vi "CRYInsert Result.vi"(8 "sOptionUpdate":string, 9 "sOption":string, 10 "Index":i32[](array[numeric]), 11 "Result":T1 {"Margin" format="%.2f"}) -> (2 "Inserted Index":i32[](array[numeric]), 3 "Inserted Name Out":string[](array[string]))   [LabVIEW 2013]
uses:
  CRYSystem/Typedef Control/CRYResult Cluster Array.ctl
  CRYSystem/Typedef Control/CRYResult Cluster.ctl
  Global/CRYCurve Library Global.vi
  Global/CRYCurves Array Global.vi
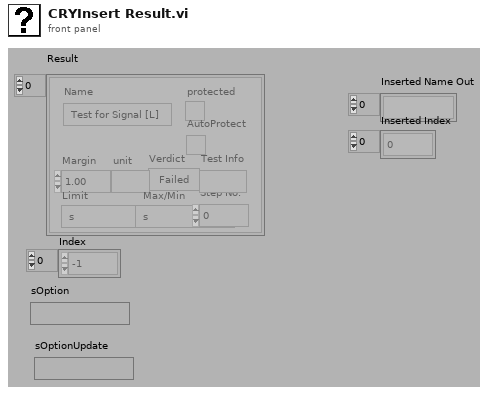
[diagram p1: front panel]
types:
  T1 = typedef "CRYResult Cluster Array.ctl" = T2[]
  T2 = typedef "CRYResult Cluster.ctl" = cluster{"Name":string, "Margin":dbl, "unit":string, "Verdict":bool, "Limit":string, "Max/Min":string, "protected":bool, "Step No.":i32, "Test Info":string, "AutoProtect":bool}
  T3 = cluster{"CurveOld":string[], "ValueOld":string[], "ResultOld":string[], "WFMOld":string[], "CurveNew":string[], "ValueNew":string[], "ResultNew":string[], "WFMNew":string[]}
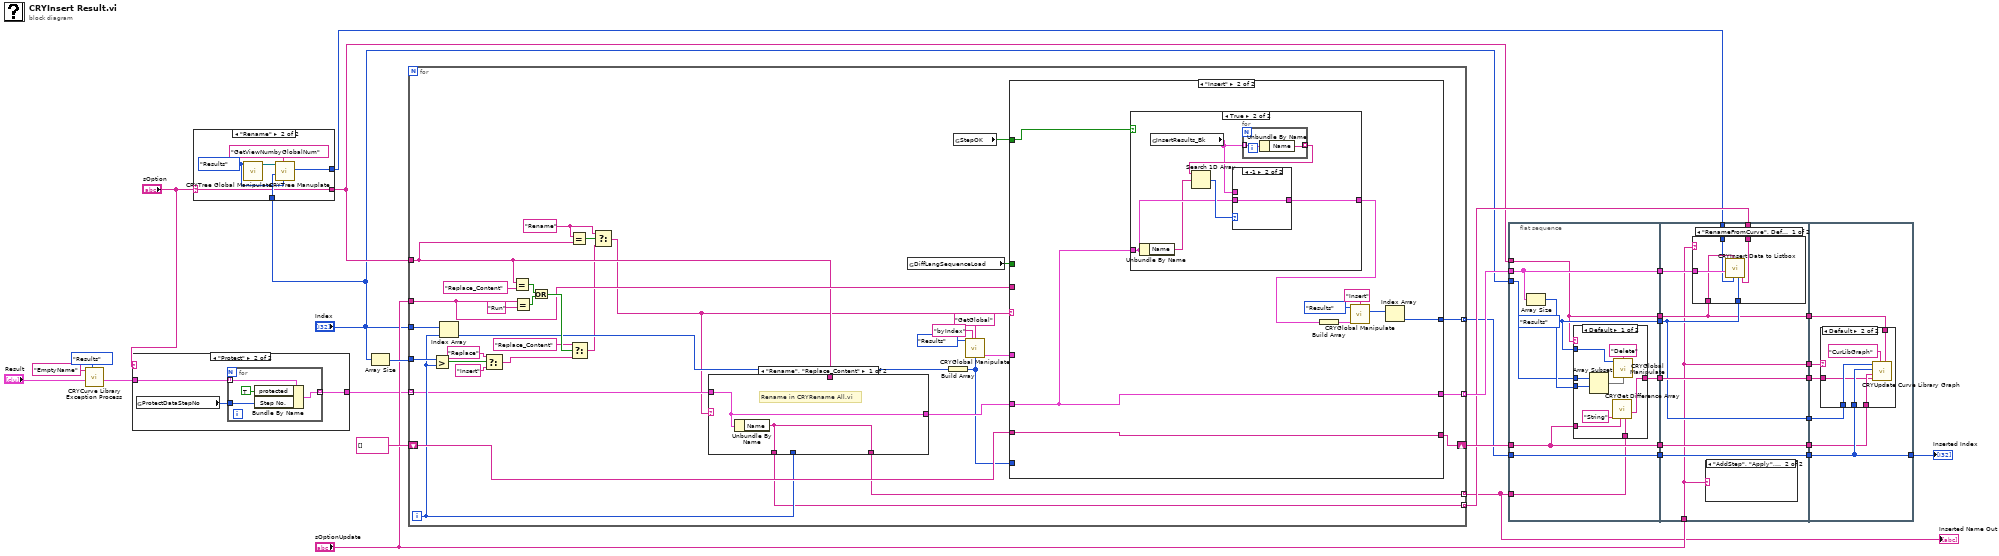
[diagram p0: block diagram]
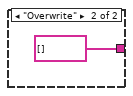
[diagram p4: hidden frame]
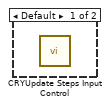
[diagram p5: hidden frame]
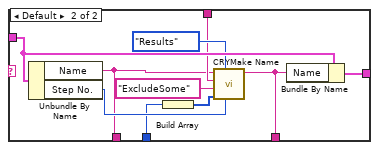
[diagram p8: hidden frame]
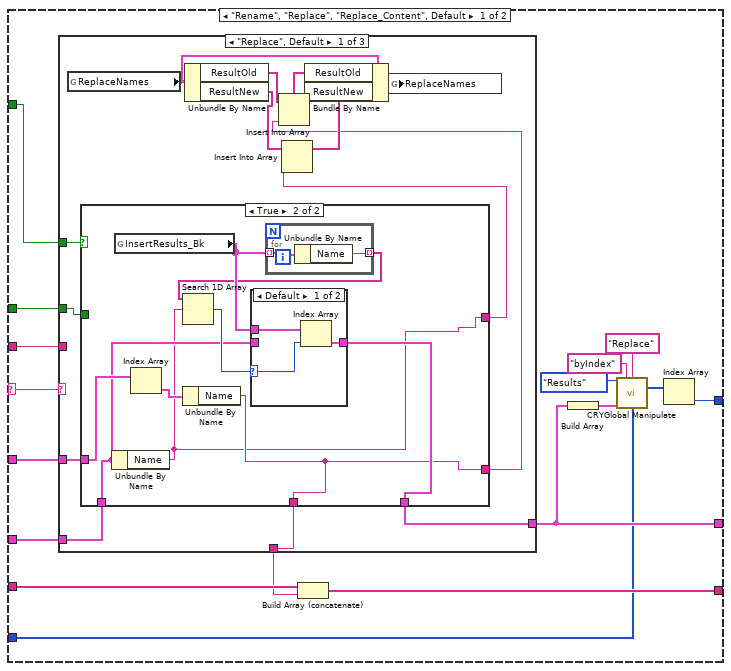
[diagram p9: hidden frame]
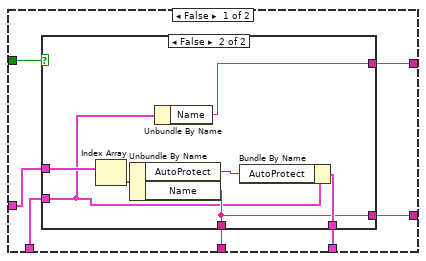
[diagram p10: hidden frame]
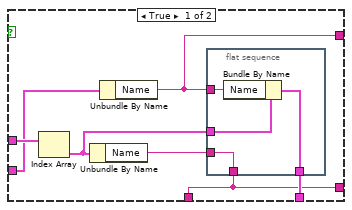
[diagram p11: hidden frame]
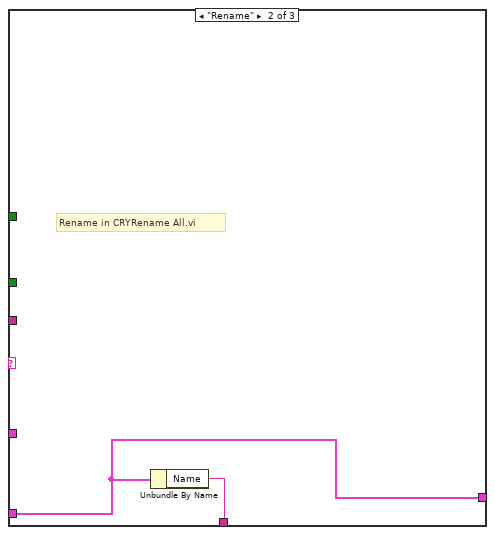
[diagram p13: hidden frame]
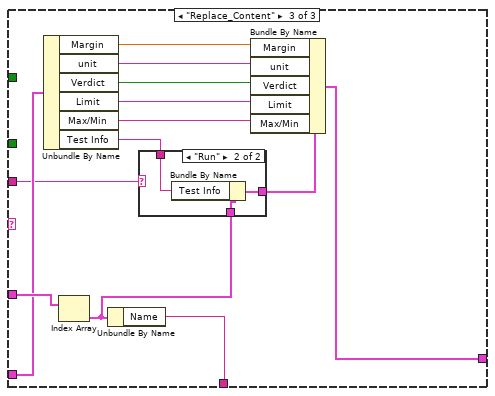
[diagram p14: hidden frame]
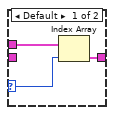
[diagram p17: hidden frame]
diagram:
  n1 = call "CRYCurve Library Exception Process.vi"("Type In"=enum16{"Curves", "Values", "Results", "WFM"}."Results", "Result"="Result", "sAction"="EmptyName") -> ("Result Out"=w1:T1)  [unwired: 6 in, 2 out]
  n2 = case shown="\"Protect\"" "sOption" {
    tunnel: w1 -> [w31 w34]
    tunnel: [w31 w33] -> w7
    frame Default {
    }
    frame "Protect" {
      n3 = global read "CRYCurve Library Global.vi" "ProtectDataStepNo"() -> (w32:i32)
      n4 = for {
        tunnel: w34 -> [w38] mode=indexing
        tunnel: [w37] -> w33 mode=indexing
        tunnel: w32 -> [w35]
        n5 = Bundle By Name(cluster=w38, "protected"=TRUE, "Step No."=w35) -> (w37:T2)
      }
    }
  }
  n6 = case shown="\"Rename\"" "sOption" {
    selector: "sOption" -> [w39 w41]
    tunnel: "Index" -> [_ w42]
    tunnel: [_ w43] -> w9
    tunnel: [w39 w41] -> w11
    frame Default {
    }
    frame "Rename" {
      w40 = enum16{"Curves", "Values", "Results", "WFM"}."Results" ("Type In")
      n7 = call "CRYTree Global Manipulate.vi"("Type In"=w40) -> ("Tree/Curve Tree"=w44:refnum<vi>)  [unwired: 7 in, 3 out]
      n8 = call "CRYTree Manuplate.vi"("Type"=w40, "sAction"="GetViewNumbyGlobalNum", "nData"=w42, "Tree in"=w44) -> ("nData Out"=w43:i32[])  [unwired: 4 in, 3 out]
    }
  }
  n9 = Array Size(array="Index") -> (size(s)=w18:i32)
  n10 = for {
    tunnel: [w71] -> w5 mode=indexing
    tunnel: "Index" -> [w70]
    tunnel: w7 -> [w61] mode=indexing
    tunnel: [w76] -> w29 mode=indexing
    tunnel: w18 -> [w79]
    shift-right: [w77] -> w28
    shift-left: string[] [] -> [w78]
    tunnel: w11 -> [w51]
    tunnel: "sOptionUpdate" -> [w62]
    tunnel: [w54] -> w12 mode=indexing
    tunnel: [w47] -> w6 mode=indexing
    i -> [w69]
    w53 = "Rename" ("y")
    n11 = Greater?(x=w79, y=w69) -> (0:w73:bool)
    n12 = Index Array(array=w70, index=w69) -> (element=w56:i32)
    n13 = Select(t="Replace" ("sOption"), s=w73, f="Insert" ("sOption")) -> (s? t:f=w72:string)
    n14 = Equal?(x=w51, y="Replace_Content") -> (x = y?=w66:bool)
    n15 = Equal?(x=w62, y="Run") -> (x = y?=w65:bool)
    n16 = Or(x=w66, y=w65) -> (x .or. y?=w64:bool)
    n17 = Equal?(x=w53, y=w51) -> (x = y?=w52:bool)
    n18 = Select(t="Replace_Content" ("y"), s=w64, f=w72) -> (s? t:f=w50:string)
    n19 = Select(t=w53, s=w52, f=w50) -> (s? t:f=w49:string)
    n20 = case shown="\"Rename\", \"Replace_Content\"" w49 {
      tunnel: [w82 w92] -> w80
      tunnel: w61 -> [w82 w91]
      tunnel: [w81 w90] -> w71
      tunnel: w69 -> [_ w85]
      tunnel: w51 -> [_ w84]
      tunnel: [w81 w83] -> w54
      frame "Rename", "Replace_Content" {
        # "Rename in CRYRename All.vi"
        n21 = Unbundle By Name(w82) -> ("Name"=w81:string)
      }
      frame Default {
        n22 = Unbundle By Name(w91) -> ("Name"=w83:string, "Step No."=w86:i32)
        n23 = Build Array(w85) -> (w88:i32[])
        n24 = call "CRYMake Name.vi"("Step No."=w86, "Type"=enum16{"Curves", "Values", "Results", "WFM"}."Results", "nData"=w88, "sOption"="ExcludeSome", "sAction"=w84, "Name In"=w83) -> ("Name Out"=w90:string)  [unwired: 4 in, 1 out]
        n25 = Bundle By Name(cluster=w91, "Name"=w90) -> (w92:T2)
      }
    }
    n26 = global read "CRYCurve Library Global.vi" "DiffLangSequenceLoad"() -> (w48:bool)
    n27 = Build Array(w56) -> (w57:i32[])
    n28 = global read "CRYCurve Library Global.vi" "StepOK"() -> (w46:bool)
    n29 = call "CRYGlobal Manipulate.vi"("Type"=enum16{"Curves", "Values", "Results", "WFM"}."Results", "sOption"="byIndex", "sAction"="GetGlobal", "nData"=w57) -> ("Results Out"=w60:T2[])  [unwired: 5 in, 6 out]
    n30 = case shown="\"Insert\"" w49 {
      selector: w49 -> [w104 _]
      tunnel: w60 -> [w108 _]
      tunnel: w80 -> [w109 w184]
      tunnel: [w106 w191] -> w77
      tunnel: w78 -> [w107 w191]
      tunnel: [w100 w184] -> w76
      tunnel: w62 -> [w103 _]
      tunnel: w57 -> [w98 _]
      tunnel: w48 -> [w96 _]
      tunnel: [w94 w186] -> w47
      tunnel: w46 -> [w93 w185]
      frame "Rename", "Replace", "Replace_Content", Default {
        n31 = case shown="\"Replace\", Default" w104 {
          tunnel: w109 -> [w119 w164 w175]
          tunnel: w108 -> [w123 _ w178]
          tunnel: [w122 w165 w177] -> w105
          tunnel: [w121 w164 w176] -> w100
          tunnel: w103 -> [_ _ w169]
          tunnel: w96 -> [w120 _ _]
          tunnel: w93 -> [w110 _ _]
          frame "Replace", Default {
            n32 = global read "CRYCurve Library Global.vi" "ReplaceNames"() -> (w118:T3)
            n33 = case shown="True" w110 {
              tunnel: w123 -> [w130 w153]
              tunnel: [w129 w150] -> w122
              tunnel: [w128 w151] -> w121
              tunnel: w120 -> [w127 _]
              tunnel: w119 -> [w126 w152]
              tunnel: [w125 w149] -> w112
              tunnel: [w124 w150] -> w111
              frame False {
                n34 = case shown="False" w127 {
                  tunnel: w130 -> [w137 w147]
                  tunnel: [w132 w143] -> w129
                  tunnel: [w136 w145] -> w128
                  tunnel: w126 -> [w135 w142]
                  tunnel: [w132 w143] -> w124
                  tunnel: [w131 w144] -> w125
                  frame True {
                    n35 = Index Array(array=w137) -> (element=w134:T2)  [unwired: 1 in]
                    n36 = Unbundle By Name(w134) -> ("Name"=w133:string)
                    n37 = Unbundle By Name(w135) -> ("Name"=w131:string)
                    n38 = flat-sequence {
                      tunnel: [w141] -> w136
                      tunnel: w134 -> [w140]
                      tunnel: w131 -> [w139]
                      tunnel: w133 -> [w138]
                      tunnel: [w138] -> w132
                      frame #0 {
                        n39 = Bundle By Name(cluster=w140, "Name"=w139) -> (w141:T2)
                      }
                    }
                  }
                  frame False {
                    n40 = Index Array(array=w147) -> (element=w148:T2)  [unwired: 1 in]
                    n41 = Unbundle By Name(w148) -> ("AutoProtect"=w146:bool, "Name"=w143:string)
                    n42 = Unbundle By Name(w142) -> ("Name"=w144:string)
                    n43 = Bundle By Name(cluster=w142, "AutoProtect"=w146) -> (w145:T2)
                  }
                }
              }
              frame True {
                n44 = Unbundle By Name(w152) -> ("Name"=w149:string)
                n45 = global read "CRYCurves Array Global.vi" "InsertResults_Bk"() -> (w156:T1)
                n46 = Index Array(array=w153) -> (element=w157:T2)  [unwired: 1 in]
                n47 = Unbundle By Name(w157) -> ("Name"=w150:string)
                n48 = for {
                  tunnel: w156 -> [w163] mode=indexing
                  tunnel: [w162] -> w154 mode=indexing
                  n49 = Unbundle By Name(w163) -> ("Name"=w162:string)
                }
                n50 = Search 1D Array(1D array=w154, element=w149) -> (index of element=w155:i32)  [unwired: 1 in]
                n51 = case shown="Default" w155 {
                  selector: w155 -> [w159 _]
                  tunnel: w156 -> [w160 _]
                  tunnel: [w158 w161] -> w151
                  tunnel: w152 -> [_ w161]
                  frame Default {
                    n52 = Index Array(array=w160, index=w159) -> (element=w158:T2)
                  }
                  frame -1 {
                  }
                }
              }
            }
            n53 = Unbundle By Name(w118) -> ("ResultOld"=w116:string[], "ResultNew"=w115:string[])
            n54 = Insert Into Array(array=w116, new element=w111) -> (w114:string[])  [unwired: 1 in]
            n55 = Insert Into Array(array=w115, new element=w112) -> (w113:string[])  [unwired: 1 in]
            n56 = Bundle By Name(cluster=w118, "ResultOld"=w114, "ResultNew"=w113) -> (w117:T3)
            n57 = global write "CRYCurve Library Global.vi" "ReplaceNames"(w117) -> ()
          }
          frame "Rename" {
            # "Rename in CRYRename All.vi"
            n58 = Unbundle By Name(w164) -> ("Name"=w165:string)
          }
          frame "Replace_Content" {
            n59 = Unbundle By Name(w175) -> ("Margin"=w174:dbl, "unit"=w173:string, "Verdict"=w172:bool, "Limit"=w171:string, "Max/Min"=w170:string, "Test Info"=w168:string)
            n60 = Index Array(array=w178) -> (element=w167:T2)  [unwired: 1 in]
            n61 = Unbundle By Name(w167) -> ("Name"=w177:string)
            n62 = case shown="\"Run\"" w169 {
              tunnel: w167 -> [w179 w182]
              tunnel: [w179 w181] -> w166
              tunnel: w168 -> [_ w180]
              frame Default {
              }
              frame "Run" {
                n63 = Bundle By Name(cluster=w182, "Test Info"=w180) -> (w181:T2)
              }
            }
            n64 = Bundle By Name(cluster=w166, "Margin"=w174, "unit"=w173, "Verdict"=w172, "Limit"=w171, "Max/Min"=w170) -> (w176:T2)
          }
        }
        n65 = Build Array (concatenate)(w107, w105) -> (w106:string[])
        n66 = Build Array(w100) -> (w99:T2[])
        n67 = call "CRYGlobal Manipulate.vi"("Type"=enum16{"Curves", "Values", "Results", "WFM"}."Results", "sOption"="byIndex", "sAction"="Replace", "Results"=w99, "nData"=w98) -> ("nData out"=w95:i32[])  [unwired: 4 in, 6 out]
        n68 = Index Array(array=w95) -> (element=w94:i32)  [unwired: 1 in]
      }
      frame "Insert" {
        n69 = case shown="True" w185 {
          tunnel: w184 -> [w192 w195]
          tunnel: [w192 w194] -> w183
          frame False {
          }
          frame True {
            n70 = Unbundle By Name(w195) -> ("Name"=w193:string)
            n71 = global read "CRYCurves Array Global.vi" "InsertResults_Bk"() -> (w196:T1)
            n72 = for {
              tunnel: w196 -> [w204] mode=indexing
              tunnel: [w203] -> w198 mode=indexing
              n73 = Unbundle By Name(w204) -> ("Name"=w203:string)
            }
            n74 = Search 1D Array(1D array=w198, element=w193) -> (index of element=w197:i32)  [unwired: 1 in]
            n75 = case shown="-1" w197 {
              selector: w197 -> [w200 _]
              tunnel: w196 -> [w201 _]
              tunnel: [w199 w202] -> w194
              tunnel: w195 -> [_ w202]
              frame Default {
                n76 = Index Array(array=w201, index=w200) -> (element=w199:T2)
              }
              frame -1 {
              }
            }
          }
        }
        n77 = Build Array(w183) -> (w188:T2[])
        n78 = call "CRYGlobal Manipulate.vi"("Type"=enum16{"Curves", "Values", "Results", "WFM"}."Results", "sAction"="Insert", "Results"=w188) -> ("nData out"=w187:i32[])  [unwired: 6 in, 6 out]
        n79 = Index Array(array=w187) -> (element=w186:i32)  [unwired: 1 in]
      }
    }
  }
  "Inserted Name Out" <- w5
  n80 = flat-sequence {
    tunnel: [w213] -> w30
    tunnel: w29 -> [w213]
    tunnel: "Index" -> [w210]
    tunnel: w28 -> [w206]
    tunnel: [w212] -> w27
    tunnel: [w206] -> w26
    tunnel: [w209] -> w23
    tunnel: [w208] -> w20
    tunnel: w6 -> [w208]
    tunnel: w11 -> [w207]
    tunnel: [w207] -> w14
    tunnel: w5 -> [w205]
    tunnel: [w230] -> w25
    tunnel: [w232] -> w24
    tunnel: w26 -> [w232]
    tunnel: w27 -> [w230]
    tunnel: w30 -> [w231]
    tunnel: w23 -> [w228]
    tunnel: [w228] -> w22
    tunnel: w20 -> [w229]
    tunnel: [w229] -> w19
    tunnel: [w224] -> w16
    tunnel: [w226] -> w15
    tunnel: w14 -> [w226]
    tunnel: "sOptionUpdate" -> [w224]
    tunnel: w12 -> [w227]
    tunnel: w9 -> [w225]
    tunnel: w25 -> [w240]
    tunnel: w24 -> [w241]
    tunnel: w22 -> [w243]
    tunnel: w19 -> [w242]
    tunnel: w16 -> [w239]
    tunnel: w15 -> [w238]
    tunnel: [w242] -> w17
    frame #0 {
      w209 = enum16{"Curves", "Values", "Results", "WFM"}."Results" ("Type")
      n81 = Array Size(array=w213) -> (size(s)=w211:i32)
      n82 = case shown="Default" w207 {
        tunnel: [w214 string[] [] ("Deleted Names")] -> w212
        tunnel: w211 -> [w222 _]
        tunnel: w210 -> [w221 _]
        tunnel: w209 -> [w219 _]
        tunnel: w206 -> [w216 _]
        tunnel: w205 -> [w215 _]
        frame Default {
          n83 = Array Subset(array=w221, index=w222) -> (w218:i32[])  [unwired: 1 in]
          n84 = call "CRYGet Difference Array.vi"("String2"=w215, "String1"=w216, "sOption"="String") -> ("StringDiff Out"=w214:string[])  [unwired: 7 in, 1 out]
          n85 = call "CRYGlobal Manipulate.vi"("Type"=w219, "sAction"="Delete", "nData"=w218) -> ()  [unwired: 6 in, 7 out]
        }
        frame "Overwrite" {
        }
      }
    }
    frame #1 {
      n86 = case shown="\"RenameFromCurve\", Default" w224 {
        tunnel: w231 -> [w237 _]
        tunnel: w228 -> [w236 _]
        tunnel: w227 -> [w235 _]
        tunnel: w226 -> [w234 _]
        tunnel: w225 -> [w233 _]
        frame "RenameFromCurve", Default {
          n87 = call "CRYInsert Data to Listbox.vi"("OrgNames"=w235, "Type"=w236, "nData"=w233, "sOption"=w234, "Results"=w237) -> ()  [unwired: 6 in, 1 out]
        }
        frame "Run" {
        }
      }
      n88 = case shown="\"AddStep\", \"Apply\", \"Run\"" w224 {
        frame Default {
          n89 = call "CRYUpdate Steps Input Control.vi"() -> ()  [unwired: 12 in]
        }
        frame "AddStep", "Apply", "Run" {
        }
      }
    }
    frame #2 {
      n90 = case shown="Default" w239 {
        tunnel: w243 -> [_ w248]
        tunnel: w242 -> [_ w247]
        tunnel: w241 -> [_ w246]
        tunnel: w240 -> [_ w245]
        tunnel: w238 -> [_ w244]
        frame "RenameFromCurve", "Run" {
        }
        frame Default {
          n91 = call "CRYUpdate Curve Library Graph.vi"("sOption 2"=w244, "sOption 1"="CurLibGraph" ("sOption"), "Deleted Names"=w245, "Replaced Old Names"=w246, "Index"=w247, "Type"=w248) -> ()  [unwired: 6 in]
        }
      }
    }
  }
  "Inserted Index" <- w17
